vi "DefaultPersonality_5775_FPGA.vi"() -> ()   [LabVIEW 2018, in "GettingStarted_5775_FPGA.lvlib"]
uses:
  GettingStarted_5775_FPGA.lvlib
  <instrlib>/_niInstr/Streaming/v1/Common/Stream State.ctl
  <vilib>/Platform/TimedLoop/XDataNode/timing_clust.ctl
  <vilib>/Platform/TimedLoop/XDataNode/nitl_modes.ctl
  <vilib>/Platform/TimedLoop/XDataNode/wakeup.ctl
  <instrlib>/FlexRIO/DRAM FIFO/v2/FPGA/DRAM FIFO/FIFO Depth.ctl
  <instrlib>/FlexRIO/API/FPGA/v1/Types/Start Trigger IO Resources.ctl
  <vilib>/rvi/Emulation/niFpgaSctlEmulationGetInTimedLoop.vi
  <vilib>/rvi/Emulation/niFpgaEmulationReportErrorSimple.vi
  <vilib>/rvi/Emulation/niFpgaGetClockAttributes.vi
  <vilib>/rvi/Emulation/niFpgaCriticalErrorInLSC.vi
  <vilib>/rvi/eio/common/nirviEmuTemplateMethod_errors.vi
  <vilib>/rvi/DataTransferAndStorage/Container/Common/niFpgaContainerGetUniqueNameForEmu.vi
  <vilib>/rvi/DataTransferAndStorage/Container/Common/niFpgaContainerSetEmuInfo.vi
  <vilib>/rvi/eio/common/nirviEmuReportErrorAndStop.vi
  <instrlib>/FlexRIO/DRAM FIFO/v2/FPGA/DRAM FIFO/Private/DRAM FIFO U256x2/Create 256x2 DRAM FIFO.vi
  <vilib>/rvi/Emulation/niFpgaProcessEmulError.vi
  <vilib>/rvi/DataTransferAndStorage/Container/Common/niFpgaContainerExecOnDevCompGetState.vi
  <vilib>/rvi/Emulation/niFpgaEmulationIsFPGAContextNoSignature.vi
  <instrlib>/_niInstr/Data Formatting/v1/FPGA/Private/Convert/Boolean Array to U16 Array.vi
  <vilib>/rvi/interface/RandomDataEmulation/nirviRandomDataMultiElementFPGAFIFO.vi
  <instcachedir>/0/nirviRandomDataMultiElementFPGAFIFO_6740B454F3C245F78F76ED91F73FD8DB.lvgen/nirviRandomDataMultiElementFPGAFIFO_6740B454F3C245F78F76ED91F73FD8DB_003.vi
  <vilib>/rvi/interface/RandomDataEmulation/niFpgaRandomDataHandleErrors.vi
  52314b2a-5df6-46e1-8e8c-f4aff1bd7d69.vi
  2c54fa2d-4261-47aa-8496-584149bfc8f9.vi
  5b634995-3468-47cf-b53b-988eeb0ffc75.vi
  99fe0684-b2b0-44f8-980b-587ad6a2a500.vi
  <instrlib>/_niInstr/Data Formatting/v1/FPGA/Private/Convert/U16 array to Boolean Array.vi
  <vilib>/Platform/TimedLoop/XDataNode/XDataNode.xnode
  <vilib>/eio/EIONode/EIONode.xnode
  <vilib>/rvi/LocalResourceManager/LocalResourceManager.xnode
  <vilib>/rvi/DataTransferAndStorage/Container/XNode/niFpgaContainer.xnode
  <vilib>/rvi/DataTransferAndStorage/Handshake/Emulation/niFpgaHandshakeEmulationRefIn.vi
  <vilib>/rvi/interface/RandomDataEmulation/nirviRandomDataFpgaMultiElementTemplate.vi
  <vilib>/Platform/TimedLoop/XDataNode/XDNodeRunTimeDep.lvlib
  <instrlib>/_niInstr/Streaming/v1/FPGA/niInstr Streaming v1 FPGA.lvlib
  <instrlib>/FlexRIO/API/FPGA/v1/FlexRIO API FPGA v1.lvlib
  <instrlib>/FlexRIO/DRAM FIFO/v2/FPGA/DRAM FIFO/DRAM FIFO v2 FPGA.lvclass
  <instrlib>/_niInstr/Data Formatting/v1/FPGA/niInstr Data Formatting v1 FPGA.lvlib
  <vilib>/rvi/FIFO/Fifo_Resource/niFpgaFifoEmulationRefIn.vi
  <instrlib>/FlexRIO/DRAM FIFO/v2/FPGA/DRAM FIFO/Private/DRAM FIFO U256x2/DRAM FIFO U256x2 v2 FPGA.lvclass
  <instrlib>/FlexRIO/API/FPGA/v1/IO/NI5775/FlexRIO 5775 FPGA v1.lvlib
  <instrlib>/_niInstr/Streaming/v1/Common/niInstr Streaming v1 Common.lvlib
panel:
  in  "flexrio.io.interleaving factor 0":u16=1
  out "flexrio.module.dram ready 0":bool
  in  "flexrio.buffer.fifo.reset 0":bool
  out "flexrio.module.io ready 0":bool
  out "flexrio.module.io error 0":i32
  out "flexrio.module.data valid 0":bool
  in  "flexrio.stream.channels enabled 0":u64 caption="stream.num samples 0"
  in  "flexrio.buffer.delay.clocks 0":u16=1
  in  "flexrio.buffer.delay.reset 0":bool
  in  "flexrio.trigger.analog.edge.rising 0":bool=TRUE
  in  "flexrio.trigger.analog.edge.hysteresis 0":fxp<+/-,32,1>
  in  "flexrio.trigger.analog.edge.threshold 0":fxp<+/-,32,1>
  in  "User-defined Start Trigger - AI":bool
  in  "flexrio.trigger.start.cfg 0":u16
  in  "flexrio.trigger.analog.edge.channel 0":fxp<+,2,2> format="%#_4g"
  in  "stream.num samples 0":u64
  in  "stream.request state 0":T1
  out "stream.state 0":T1
  out "stream.samples transferred 0":u64
  out "stream.metadata 0":u64
  # "Device Utilization\n---------------------------\nTotal Slices: 60.9% (18438 out of 30300)\nSlice Registers: 22.1% (107273 out of 484800)\nSlice LUTs: 36.1% (87476 out of 242400)\nBlock RAMs: 49.5% (297 out of 600)\nDSP48s: 0.3% (6 out of 1920)\n\nNote: Utilization numbers are for the KU040. Exact values will vary for the KU060 and KU035."
  # "Data Path Configuration"
  # "AI Trigger Configuration"
  # "AI Stream Configuration"
  # "Module Status"
  # "User-defined Controls"
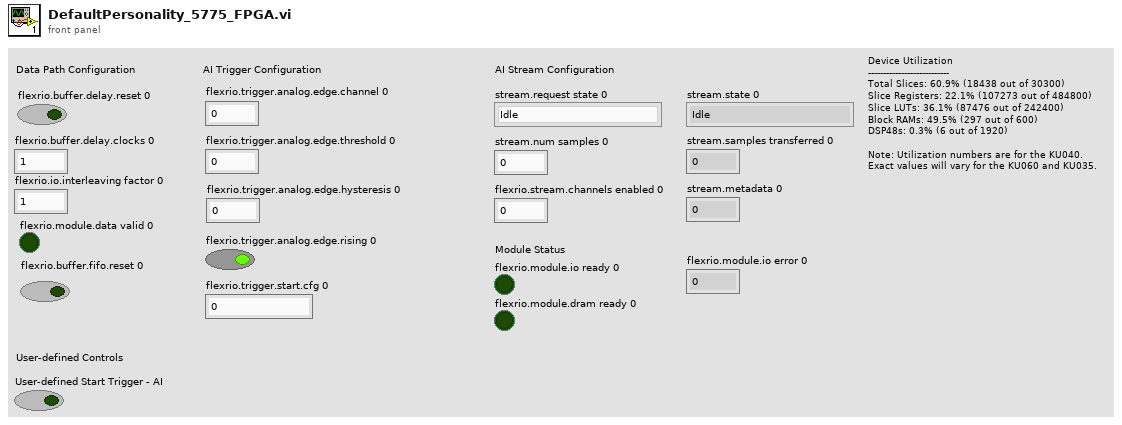
[diagram p1: front panel]
types:
  T1 = typedef "niInstr Streaming v1 Common.lvlib/Stream State.ctl" = enum8{"Idle", "Finite Transfer", "Continuous", "Done", "Error", "Not Ready", "Cancel"}
  T2 = typedef "DRAM FIFO v2 FPGA.lvclass/FIFO Depth.ctl" = u8
  T3 = typedef "XDNodeRunTimeDep.lvlib/timing_clust.ctl" = cluster{"Expected End [f-1]":u64, "Actual End [f-1]":u64, "Finished Late? [f-1]":bool, "Expected End [i-1]":u64, "Actual End [i-1]":u64, "Finished Late? [i-1]":bool, "Expected Start [i]":u64, "Actual Start [i]":u64, "Expected Start [f]":u64, "Actual Start [f]":u64, "Source Name":string, "Structure Name":string, "Period":i64, "Deadline":i64, "Offset":i64, "Start":i64, "Priority":i32, "Timeout":i32, "Mode":T4, "Wakeup Reason":T5, "Error":errorcluster, "Source Type":string, "Secondary Source Type":string, "Global End Time":u64, "Global Start Time":u64, "Frame Duration":u64, "Iteration Duration":u64, "Assigned CPU":i32, "I/O Scan Engine Mode":u32}
  T4 = typedef "XDNodeRunTimeDep.lvlib/nitl_modes.ctl" = enum32{"No Change", "Process missed periods, maintain original phase", "Discard missed periods, maintain original phase", "Process missed periods, ignore original phase", "Discard missed periods, ignore original phase"}
  T5 = typedef "XDNodeRunTimeDep.lvlib/wakeup.ctl" = enum32{"Normal", "Aborted", "Asynchronous wakeup", "Timing source error", "Timed loop error", "Timeout"}
  T6 = typedef "FlexRIO API FPGA v1.lvlib/Start Trigger IO Resources.ctl" = cluster{"start trigger":refnum<k21>, "started event":refnum<k21>, "start trigger for export":refnum<k21>, "start trigger for tclk":refnum<k21>}
  T7 = typedef "FlexRIO API FPGA v1.lvlib/Start Trigger Control.ctl" = cluster{"arm start":bool, "done":bool}
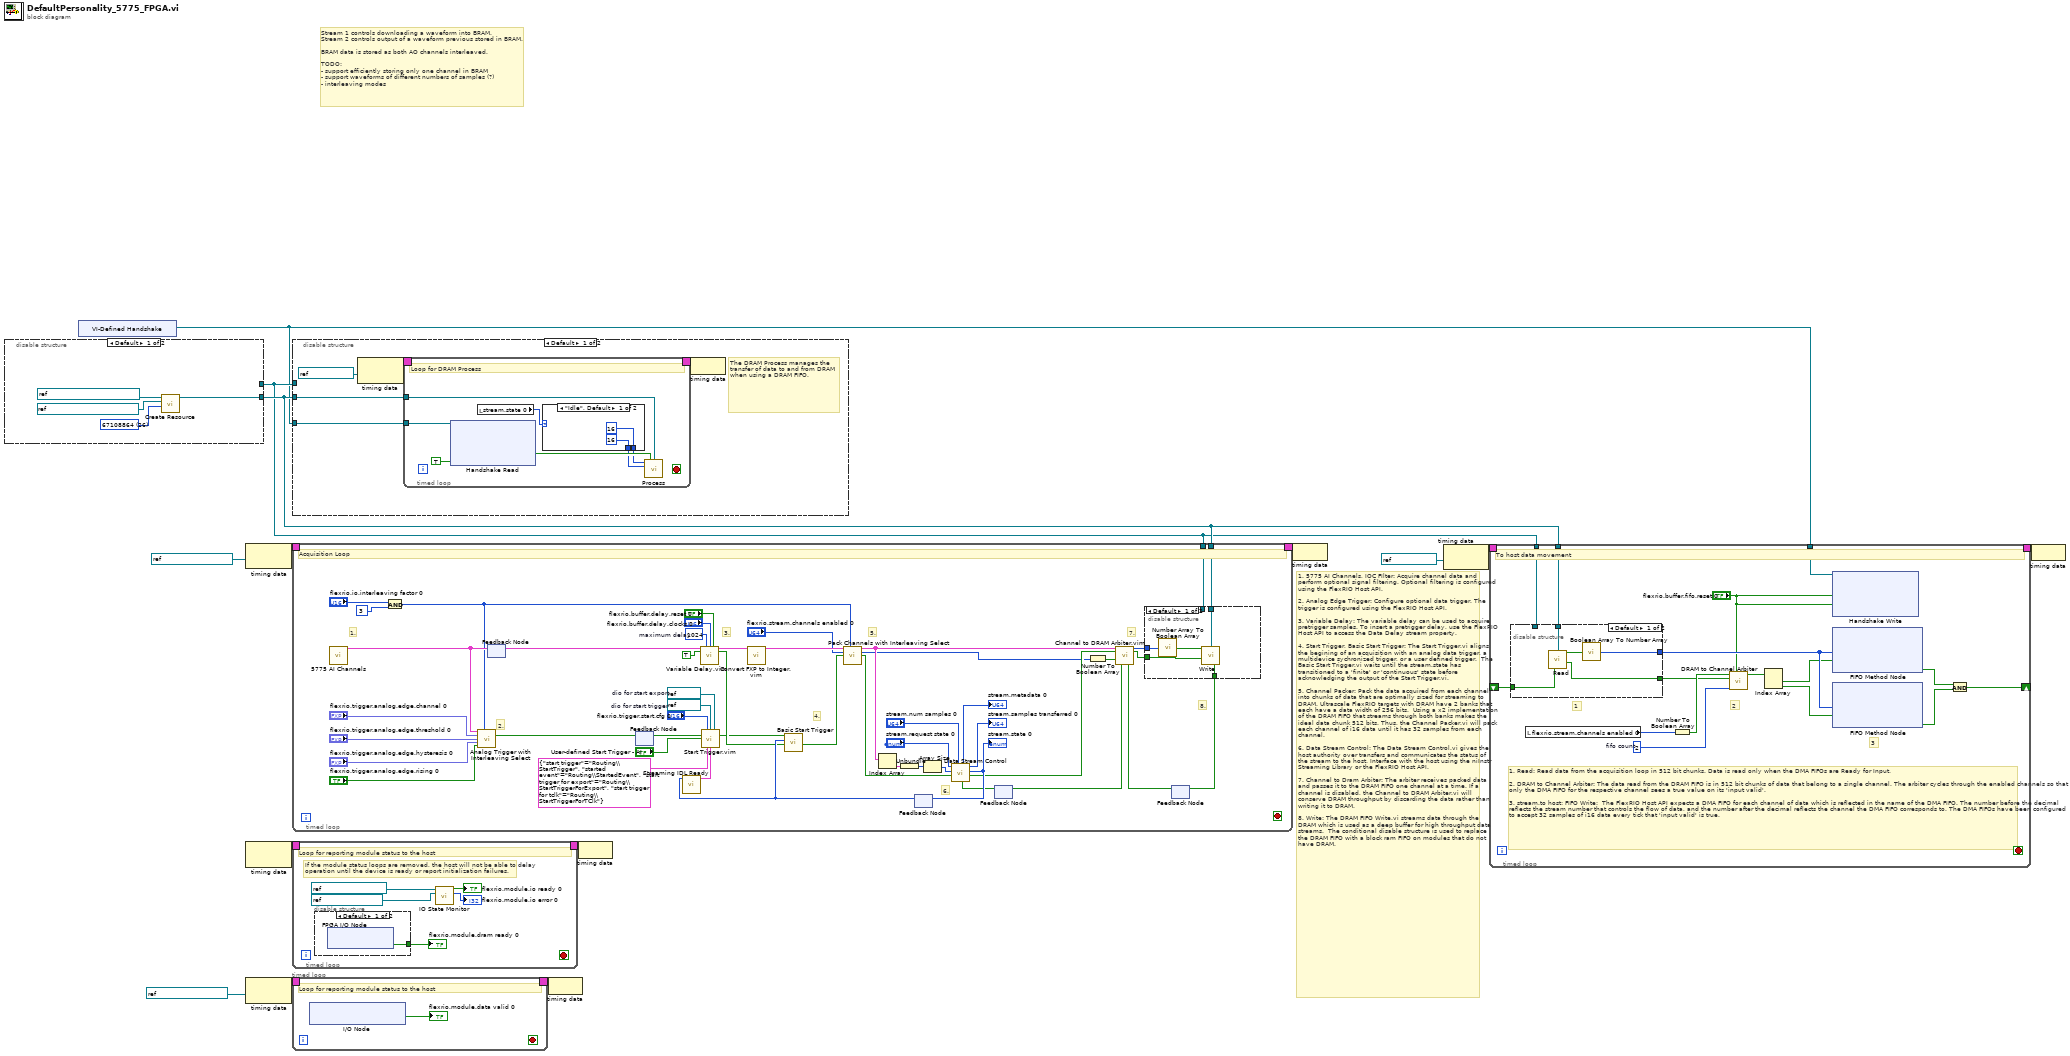
[diagram p0: block diagram]
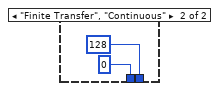
[diagram p2: hidden frame]
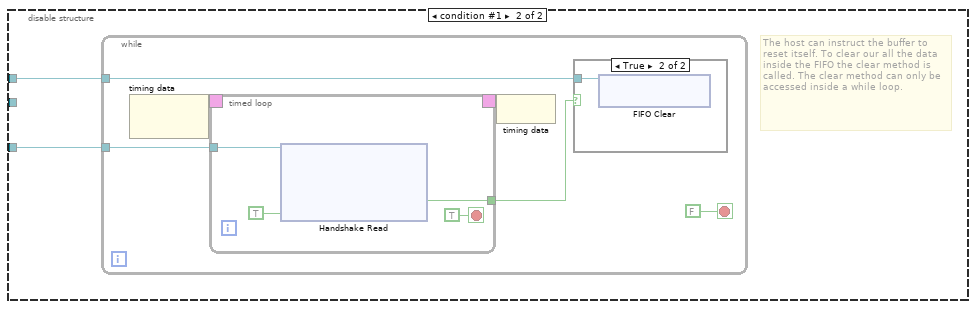
[diagram p3: hidden frame]
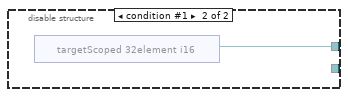
[diagram p5: hidden frame]
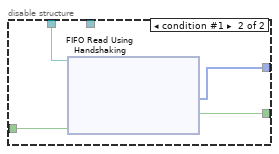
[diagram p6: hidden frame]
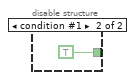
[diagram p7: hidden frame]
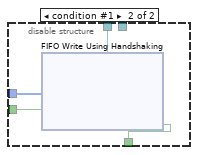
[diagram p8: hidden frame]
diagram:
  # "Stream 1 controls downloading a waveform into BRAM.\nStream 2 controls output of a waveform previous stored in BRAM.\n\nBRAM data is stored as both AO channels interleaved.\n\nTODO:\n- support efficiently storing only one channel in BRAM\n- support waveforms of different numbers of samples (?)\n- interleaving modes"
  # "1. 5775 AI Channels, IOC FIlter: Acquire channel data and perform optional signal filtering. Optional filtering is configured using the FlexRIO Host API.\n\n2. Analog Edge Trigger: Configure optional data trigger. The trigger is configured using the FlexRIO Host API.\n\n3. Variable Delay: The variable delay can be used to acquire pretrigger samples. To insert a pretrigger delay, use the FlexRIO Host API to access the Data Delay stream property. \n\n4. Start Trigger, Basic Start Trigger: The Start Trigger.vi aligns the begining of an acquisition with an analog data trigger, a multidevice sychronized trigger, or a user defined trigger.  The Basic Start Trigger.vi waits until the stream.state has transitioned to a 'finite' or 'continuous' state before acknowledging the output of the Start Trigger.vi.\n\n5. Channel Packer: Pack the data acquired from each channel into chunks of data that are optimally sized for streaming to DRAM. Ultrascale FlexRIO targets with DRAM have 2 banks that each have a data width of 256 bits.  Using a x2 implementation of the DRAM FIFO that streams through both banks makes the ideal data chunk 512 bits. Thus, the Channel Packer.vi will pack each channel of i16 data until it has 32 samples from each channel. \n\n6. Data Stream Control: The Data Stream Control.vi gives the host authority over transfers and communicates the status of the stream to the host. Interface with the host using the niInstr Streaming Library or the FlexRIO Host API. \n\n7. Channel to Dram Arbiter: The arbiter receives packed data and passes it to the DRAM FIFO one channel at a time. If a channel is disabled, the Channel to DRAM Arbiter.vi will conserve DRAM throughput by discarding the data rather than writing it to DRAM. \n\n8. Write: The DRAM FIFO Write.vi streams data through the DRAM which is used as a deep buffer for high throughput data streams.  The conditional disable structure is used to replace the DRAM FIFO with a block ram FIFO on modules that do not have DRAM."
  n1 = disable-structure shown="Default" {
    disable-tunnel: [w18 _] -> w6
    disable-tunnel: [_ w19] -> w5
    frame condition #0 (active) {
      w15 = T2 26 items=["4"=2, "8"=3, "16"=4, "32"=5, "64"=6, "128"=7, "256"=8, "512"=9, "1024"=10, "2048"=11, "4096"=12, "8192"=13, "16384"=14, "32768"=15, "65536"=16, "131072"=17, "262144"=18, "524288"=19, "1048576"=20, "2097152"=21, "4194304"=22, "8388608"=23, "16777216"=24, "33554432"=25, "67108864"=26, "134217728"=27, "268435456"=28, "536870912"=29, "1073741824"=30, "2147483648"=31, "4294967296"=32] ("actual # of DRAM elements")
      n2 = call-poly <instrlib>:"Create Resource.vi"("actual # of DRAM elements"=w15, "memory refnum 2"=refnum<k21> "DRAM FIFO Bank1 67108864" ("memory refnum"), "memory refnum"=refnum<k21> "DRAM FIFO Bank0 67108864") -> ("DRAM FIFO ref out"=w18:refnum<class "DRAM FIFO v2 FPGA.lvclass">)  [unwired: 8 in]
    }
    frame condition #1 {
      n3 = xnode "targetScoped 32element i16"() -> ("FIFO Out"=w19:refnum<k21>)
    }
  }
  n4 = xnode "VI-Defined Handshake"() -> ("Handshake Out"=w4:refnum<k21>)
  n5 = node-c288(refnum<k21> "IO Socket\\Data Clock" ("Source Name")) -> (w14:T3)
  n6 = node-c288() -> (w11:T3)  [unwired: 1 in]
  n7 = node-c288(refnum<k21> "IO Socket\\Data Clock" ("Source Name")) -> (w3:T3)
  n8 = disable-structure shown="Default" {
    disable-tunnel: w6 -> [w21 _]
    disable-tunnel: w5 -> [_ w43]
    disable-tunnel: w4 -> [w20 w42]
    frame condition #0 (active) {
      # "The DRAM Process manages the transfer of data to and from DRAM when using a DRAM FIFO."
      n9 = node-c288(refnum<k21> "DRAM Clock" ("Source Name")) -> (w24:T3)
      n10 = timed-loop {
        timing: w24 -> [_]
        timing-out: [_] -> w23
        tunnel: w21 -> [w31]
        tunnel: w20 -> [w30]
        stop <- _ stop-if-true
        # "Loop for DRAM Process"
        n11 = xnode ("Handshake Read")("Ready for Output"=TRUE, "Handshake In"=w30) -> ("Output Valid"=w28:bool)  [unwired: 2 out]
        n12 = local read "stream.state 0"() -> (w27:T1)
        n13 = case shown="\"Idle\", Default" w27 {
          tunnel: [u16 16 ("write grant time (clock ticks)") u16 128 ("write grant time (clock ticks)")] -> w26
          tunnel: [u16 16 ("read grant time (clock ticks)") u16 0 ("read grant time (clock ticks)")] -> w25
          frame "Idle", Default {
          }
          frame "Finite Transfer", "Continuous" {
          }
        }
        n14 = call <instrlib>:"Process.vi"("write grant time (clock ticks)"=w26, "reset DRAM"=w28, "DRAM FIFO ref in"=w31, "read grant time (clock ticks)"=w25) -> ()  [unwired: 10 in, 2 out]
      }
      n15 = node-c288(w23) -> ()
    }
    frame condition #1 {
      # "The host can instruct the buffer to reset itself. To clear our all the data inside the FIFO the clear method is called. The clear method can only be accessed inside a while loop."
      n16 = while {
        tunnel: w43 -> [w49]
        tunnel: w42 -> [w48]
        stop <- FALSE stop-if-true
        n17 = node-c288() -> (w45:T3)  [unwired: 1 in]
        n18 = timed-loop {
          timing: w45 -> [_]
          timing-out: [_] -> w44
          tunnel: w48 -> [w53]
          tunnel: [w51] -> w46
          stop <- TRUE stop-if-true
          n19 = xnode ("Handshake Read")("Ready for Output"=TRUE, "Handshake In"=w53) -> ("Output Valid"=w51:bool)  [unwired: 2 out]
        }
        n20 = node-c288(w44) -> ()
        n21 = case shown="True" w46 {
          tunnel: w49 -> [_ w58]
          frame False {
          }
          frame True {
            n22 = xnode ("FIFO Clear")("FIFO In"=w58) -> ()  [unwired: 1 out]
          }
        }
      }
    }
  }
  n23 = timed-loop {
    timing: w14 -> [_]
    timing-out: [_] -> w13
    tunnel: w6 -> [w80]
    tunnel: w5 -> [w79]
    stop <- _ stop-if-true
    w93 = u16 1024  # maximum delay
    w99 = refnum<k21> "DIO 0"  # dio for start trigger
    w98 = refnum<k21> "DIO 1"  # dio for start export
    # "5."
    # "2."
    # "8."
    # "7."
    # "6."
    # "4."
    # "3."
    # "1."
    # "Acquisition Loop"
    n24 = call <instrlib>:"5775 AI Channels.vi"() -> ("all channels"=w74:cluster{fxp<+/-,12,1>[]}[])  [unwired: 15 in]
    n25 = And(x="flexrio.io.interleaving factor 0", y=u16 3) -> (x .and. y?=w61:u16)
    n26 = call "Analog Trigger with Interleaving Select.vi"("all channels"=w74, "interleaving factor"=w61, "channel"="flexrio.trigger.analog.edge.channel 0", "trigger level"="flexrio.trigger.analog.edge.threshold 0", "hysteresis level"="flexrio.trigger.analog.edge.hysteresis 0", "rising edge"="flexrio.trigger.analog.edge.rising 0") -> ("triggered"=w75:bool)  [unwired: 9 in]
    n27 = feedback #1() -> (w92:cluster{fxp<+/-,12,1>[]}[])  [unwired: 1 in]
    n28 = feedback-in #1(w74) -> ()
    n29 = feedback-in #2(w75) -> ()
    n30 = feedback #2() -> (w95:bool)  [unwired: 1 in]
    n31 = call "Variable Delay.vim"("Array in"=w92, "maximum delay"=w93, "delay"="flexrio.buffer.delay.clocks 0", "reset"="flexrio.buffer.delay.reset 0", "data valid"=TRUE) -> ("Array out"=w86:cluster{fxp<+/-,12,1>[]}[], "data valid?"=w91:bool)  [unwired: 8 in, 1 out]
    n32 = call "Convert FXP to Integer.vim"("Array in"=w86) -> ("Array"=w69:cluster{i16[]}[])  [unwired: 14 in]
    n33 = feedback #3() -> (w97:T1)  [unwired: 1 in]
    n34 = call <instrlib>:"Streaming IDL Ready.vi"("stream.state"=w97) -> ("start trigger control"=w101:T7)  [unwired: 10 in]
    n35 = call "Start Trigger.vim"("flexrio.trigger.start.cfg 0"="flexrio.trigger.start.cfg 0", "dio start"=w99, "dio for start export"=w98, "analog trigger"=w95, "user-defined start trigger"="User-defined Start Trigger - AI", "trigger io resources"=T6 {"start trigger"="Routing\\StartTrigger", "started event"="Routing\\StartedEvent", "start trigger for export"="Routing\\StartTriggerForExport", "start trigger for tclk"="Routing\\StartTriggerForTClk"}, "start trigger control"=w101) -> ("conditioned start trigger"=w60:bool)  [unwired: 6 in, 2 out]
    n36 = call <instrlib>:"Basic Start Trigger.vi"("data valid?"=w91, "stream.state"=w97, "start trigger"=w60) -> ("data valid"=w67:bool)  [unwired: 8 in]
    n37 = call "Pack Channels with Interleaving Select.vi"("Array"=w69, "interleaving factor"=w61, "channels enabled"="flexrio.stream.channels enabled 0", "data valid?"=w67) -> ("Array out"=w68:cluster{i16[]}[], "channels enabled out"=w65:u64, "data valid"=w66:bool)  [unwired: 9 in]
    n38 = Index Array(array=w68) -> (element=w88:cluster{i16[]})  [unwired: 1 in]
    n39 = Unbundle(w88) -> (w87:i16[])
    n40 = Array Size(array=w87) -> (size(s)=w107:i32)
    n41 = feedback #4() -> (w76:bool)  [unwired: 1 in]
    n42 = call <instrlib>:"Data Stream Control.vi"("ready for input?"=w76, "stream.num samples 0"="stream.num samples 0", "data valid"=w66, "element count"=w107, "stream.request state 0"="stream.request state 0") -> ("send data"=w83:bool, "stream.state 0"=w102:T1, "stream.samples transferred 0"=→"stream.samples transferred 0":u64, "stream.metadata 0"=→"stream.metadata 0":u64)  [unwired: 2 in, 1 out]
    "stream.state 0" <- w102
    n43 = feedback-in #3(w102) -> ()
    n44 = Number To Boolean Array(number=w65) -> (Boolean array=w84:bool[])
    n45 = feedback #5() -> (w78:bool)  [unwired: 1 in]
    n46 = call "Channel to DRAM Arbiter.vim"("channels in"=w68, "valid in"=w83, "channels enabled"=w84, "ready for output"=w78) -> ("data"=w85:i16[], "valid out"=w81:bool, "ready for input"=w77:bool)  [unwired: 9 in]
    n47 = feedback-in #4(w77) -> ()
    n48 = disable-structure shown="Default" {
      disable-tunnel: w85 -> [w112 w115]
      disable-tunnel: [w110 w113] -> w82
      disable-tunnel: w81 -> [w109 w114]
      disable-tunnel: w80 -> [w108 _]
      disable-tunnel: w79 -> [_ w116]
      frame condition #0 (active) {
        n49 = call-poly <instrlib>:"Number Array To Boolean Array.vi"("data in"=w112) -> ("data out"=w111:bool[])  [unwired: 14 in]
        n50 = call <instrlib>:"Write.vi"("element"=w111, "DRAM FIFO ref in"=w108, "input valid"=w109) -> ("ready for input"=w110:bool)  [unwired: 12 in]
      }
      frame condition #1 {
        n51 = xnode ("FIFO Write Using Handshaking")("Element"=w115, "Input Valid"=w114, "FIFO In"=w116) -> ("Ready for Input"=w113:bool)  [unwired: 1 out]
      }
    }
    n52 = feedback-in #5(w82) -> ()
  }
  n53 = timed-loop {
    timing: w11 -> [_]
    timing-out: [_] -> w10
    stop <- _ stop-if-true
    # "If the module status loops are removed, the host will not be able to delay operation until the device is ready or report initialization failures."
    # "Loop for reporting module status to the host"
    n54 = disable-structure shown="Default" {
      disable-tunnel: [w124 TRUE ("flexrio.module.dram ready 0")] -> w121
      frame condition #0 (active) {
        n55 = xnode "FPGA I/O Node"() -> ("DRAM Ready"=w124:bool)  [unwired: 1 in, 1 out]
      }
      frame condition #1 {
      }
    }
    "flexrio.module.dram ready 0" <- w121
    n56 = call <instrlib>:"IO State Monitor.vi"("io error resource"=refnum<k21> "IO Socket\\IO Error" ("FPGA I/O In"), "io ready resource"=refnum<k21> "IO Socket\\IO Ready" ("FPGA I/O In")) -> ("flexrio.module.io error 0"=→"flexrio.module.io error 0":i32, "flexrio.module.io ready 0"=→"flexrio.module.io ready 0":bool)  [unwired: 8 in]
  }
  n57 = timed-loop {
    timing: w3 -> [_]
    timing-out: [_] -> w2
    stop <- _ stop-if-true
    # "Loop for reporting module status to the host"
    n58 = xnode "I/O Node"() -> ("IO Socket\\AI Data Valid"=→"flexrio.module.data valid 0":bool)  [unwired: 1 in, 1 out]
  }
  n59 = node-c288(w2) -> ()
  n60 = node-c288(w10) -> ()
  n61 = node-c288(w13) -> ()
  n62 = node-c288(refnum<k21> "PXIe_CLK200" ("Source Name")) -> (w9:T3)
  n63 = timed-loop {
    timing: w9 -> [_]
    timing-out: [_] -> w8
    tunnel: w6 -> [w145]
    shift-right: [w131] -> _
    shift-left: _ -> [w143]
    tunnel: w5 -> [w142]
    tunnel: w4 -> [w141]
    stop <- _ stop-if-true
    w135 = 2  # fifo count
    # "3"
    # "2"
    # "1. Read: Read data from the acquisition loop in 512 bit chunks. Data is read only when the DMA FIFOs are Ready for Input.\n\n2. DRAM to Channel Arbiter: The data read from the DRAM FIFO is in 512 bit chunks of data that belong to a single channel. The arbiter cycles through the enabled channels so that only the DMA FIFO for the respective channel sees a true value on its 'input valid'. \n\n3. stream.to host: FIFO Write:  The FlexRIO Host API expects a DMA FIFO for each channel of data which is reflected in the name of the DMA FIFO. The number before the decimal reflects the stream number that controls the flow of data, and the number after the decimal reflects the channel the DMA FIFO corresponds to. The DMA FIFOs have been configured to accept 32 samples of i16 data every tick that 'input valid' is true."
    # "1"
    # "To host data movement"
    n64 = disable-structure shown="Default" {
      disable-tunnel: w145 -> [w151 _]
      disable-tunnel: [w150 w153] -> w136
      disable-tunnel: [w149 w154] -> w144
      disable-tunnel: w143 -> [w147 w152]
      disable-tunnel: w142 -> [_ w155]
      frame condition #0 (active) {
        n65 = call <instrlib>:"Read.vi"("DRAM FIFO ref in"=w151, "ready for output"=w147) -> ("element"=w148:bool[], "output valid"=w150:bool)  [unwired: 12 in]
        n66 = call-poly <instrlib>:"Boolean Array To Number Array.vi"("data in"=w148) -> ("data out"=w149:u16[])  [unwired: 14 in]
      }
      frame condition #1 {
        n67 = xnode ("FIFO Read Using Handshaking")("Ready for Output"=w152, "FIFO In"=w155) -> ("Element"=w154:i16[], "Output Valid"=w153:bool)  [unwired: 1 out]
      }
    }
    n68 = local read "flexrio.stream.channels enabled 0"() -> (w146:u64)
    n69 = Number To Boolean Array(number=w146) -> (Boolean array=w137:bool[])
    n70 = call <instrlib>:"DRAM to Channel Arbiter.vi"("reset"="flexrio.buffer.fifo.reset 0", "channel count"=w135, "input valid"=w136, "channels enabled"=w137) -> ("valid channel"=w140:bool[])  [unwired: 6 in, 1 out]
    n71 = Index Array(array=w140) -> (element #1=w139:bool, element #2=w138:bool)  [unwired: 2 in]
    n72 = xnode ("Handshake Write")("Data"="flexrio.buffer.fifo.reset 0", "Input Valid"="flexrio.buffer.fifo.reset 0", "Handshake In"=w141) -> ()  [unwired: 2 out]
    n73 = xnode ("FIFO Method Node")("Element"=w144, "Input Valid"=w139) -> ("Ready for Input"=w133:bool)  [unwired: 1 in, 1 out]
    n74 = xnode ("FIFO Method Node")("Element"=w144, "Input Valid"=w138) -> ("Ready for Input"=w132:bool)  [unwired: 1 in, 1 out]
    n75 = And(x=w133, y=w132) -> (x .and. y?=w131:bool)
  }
  n76 = node-c288(w8) -> ()
